vi "Load TabAcqType index.vi"(8 "error in (no error)":errorcluster, 11 "S4GUI in":refnum<class "S4GUI.lvclass">) -> (0 "error out":errorcluster, 3 "S4GUI out":refnum<class "S4GUI.lvclass">)   [LabVIEW 2018, in "S4GUI.lvclass"]
uses:
  S4GUI.lvclass
  S4GUI.lvclass/S4GUI.ctl
  <vilib>/Utility/config.llb/Read Key (U32).vi
  Publisher/Publisher.lvclass
  <vilib>/Utility/config.llb/NI_LVConfig.lvlib
panel:
  out "file created?":bool
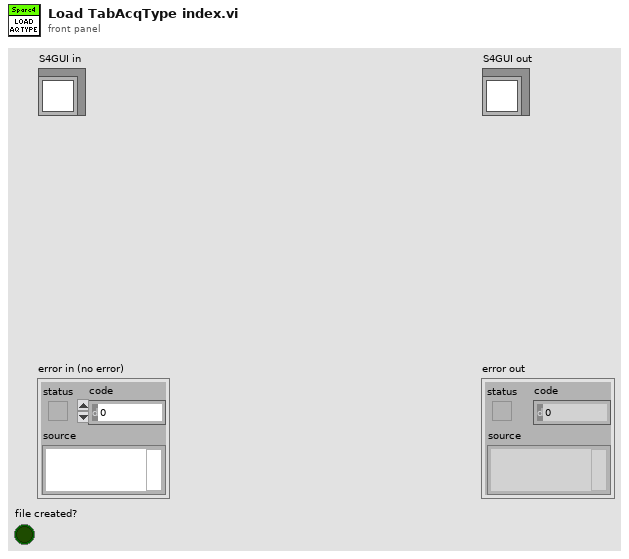
[diagram p1: front panel]
types:
  T1 = typedef "NI_LVConfig.lvlib/Config Data RefNum.ctl" = refnum<k1>
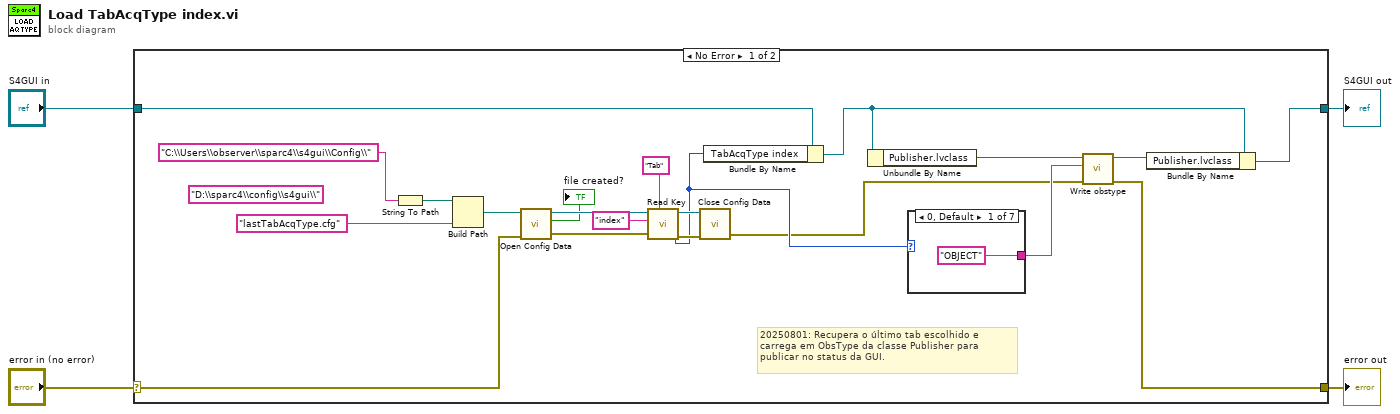
[diagram p0: block diagram]
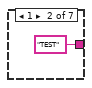
[diagram p2: hidden frame]
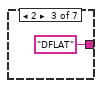
[diagram p3: hidden frame]
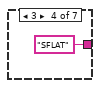
[diagram p4: hidden frame]
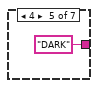
[diagram p5: hidden frame]
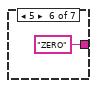
[diagram p6: hidden frame]
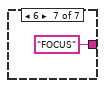
[diagram p7: hidden frame]
diagram:
  n1 = case shown="No Error" "error in (no error)" {
    selector: "error in (no error)" -> [w16 w34]
    tunnel: [w5 w34] -> w3
    tunnel: [w10 w33] -> w1
    tunnel: "S4GUI in" -> [w14 w33]
    frame No Error {
      (unwired) "D:\\sparc4\\config\\s4gui\\" ("string")
      # "20250801: Recupera o último tab escolhido e carrega em ObsType da classe Publisher para publicar no status da GUI."
      n2 = String To Path(string="C:\\Users\\observer\\sparc4\\s4gui\\Config\\") -> (path=w18:path)
      n3 = Build Path(base path=w18, name or relative path="lastTabAcqType.cfg") -> (appended path=w25:path)
      n4 = call <vilib>:"Open Config Data.vi"("error in (no error)"=w16, "configuration file path"=w25) -> ("error out"=w22:errorcluster, "file created?"=→"file created?":bool, "refnum"=w24:T1)  [unwired: 7 in]
      n5 = call-poly <vilib>:"Read Key.vi"("section"="Tab", "error in (no error)"=w22, "key"="index", "refnum"=w24) -> ("error out"=w19:errorcluster, "value"=w12:u32, "refnum out"=w20:T1)  [unwired: 4 in, 1 out]
      n6 = call <vilib>:"Close Config Data.vi"("error in (no error)"=w19, "refnum"=w20) -> ("error out"=w6:errorcluster)  [unwired: 8 in, 1 out]
      n7 = Bundle By Name(cluster=w14, "TabAcqType index"=w12) -> (w11:refnum<class "S4GUI.lvclass">)
      n8 = Unbundle By Name(w11) -> ("Publisher.lvclass"=w9:refnum<class "Publisher.lvclass">)
      n9 = case shown="0, Default" w12 {
        tunnel: ["OBJECT" ("section") "TEST" ("section") "DFLAT" ("section") "SFLAT" ("section") "DARK" ("section") "ZERO" ("section") "FOCUS" ("section")] -> w7
        frame 0, Default {
        }
        frame 1 {
        }
        frame 2 {
        }
        frame 3 {
        }
        frame 4 {
        }
        frame 5 {
        }
        frame 6 {
        }
      }
      n10 = call-dynamic "Write obstype.vi"("error in (no error)"=w6, "obstype"=w7, "Publisher in"=w9) -> ("error out"=w5:errorcluster, "Publisher out"=w8:refnum<class "Publisher.lvclass">)  [unwired: 7 in]
      n11 = Bundle By Name(cluster=w11, "Publisher.lvclass"=w8) -> (w10:refnum<class "S4GUI.lvclass">)
    }
    frame Error {
    }
  }
  "error out" <- w3
  "S4GUI out" <- w1
